vi "Escritura_Ingen.vi"(10 "Entrada_Variables":u16[](array[numeric])) -> (2 "Escritura_Variabes":u16[](array[numeric]))   [LabVIEW 2017, in "Lib_Esclavo_Ingen.lvlib"]
uses:
  Lib_Esclavo_Ingen.lvlib
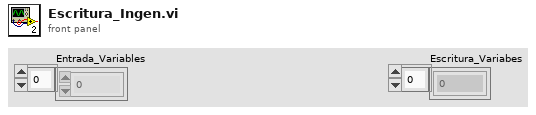
[diagram p1: front panel]
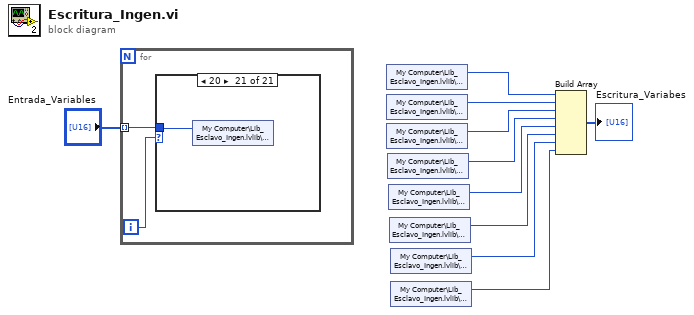
[diagram p0: block diagram]
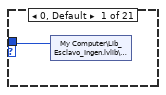
[diagram p2: hidden frame]
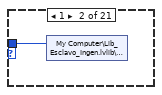
[diagram p3: hidden frame]
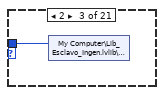
[diagram p4: hidden frame]
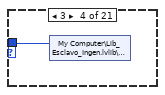
[diagram p5: hidden frame]
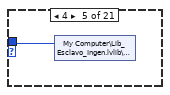
[diagram p6: hidden frame]
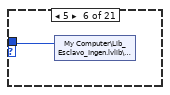
[diagram p7: hidden frame]
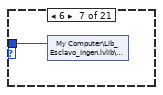
[diagram p8: hidden frame]
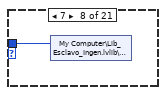
[diagram p9: hidden frame]
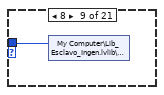
[diagram p10: hidden frame]
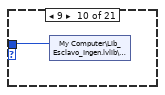
[diagram p11: hidden frame]
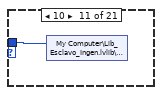
[diagram p12: hidden frame]
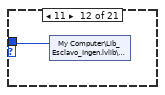
[diagram p13: hidden frame]
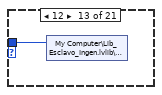
[diagram p14: hidden frame]
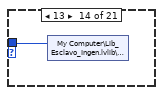
[diagram p15: hidden frame]
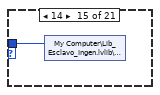
[diagram p16: hidden frame]
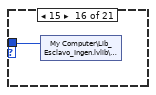
[diagram p17: hidden frame]
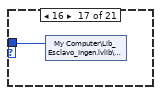
[diagram p18: hidden frame]
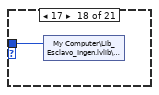
[diagram p19: hidden frame]
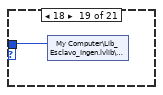
[diagram p20: hidden frame]
diagram:
  n1 = for {
    tunnel: "Entrada_Variables" -> [w11] mode=indexing
    i -> [w12]
    n2 = case shown="20" w12 {
      tunnel: w11 -> [w13 w14 w15 w16 w17 w18 w19 w20 w21 w22 w23 w24 w25 w26 w27 w28 w29 w30 w31 w32 w33]
      frame 0, Default {
        n3 = shared-variable "My Computer\\Lib_Esclavo_Ingen.lvlib\\300001"(w13) -> ()  [unwired: 1 in, 1 out]
      }
      frame 1 {
        n4 = shared-variable "My Computer\\Lib_Esclavo_Ingen.lvlib\\300002"(w14) -> ()  [unwired: 1 in, 1 out]
      }
      frame 2 {
        n5 = shared-variable "My Computer\\Lib_Esclavo_Ingen.lvlib\\300003"(w15) -> ()  [unwired: 1 in, 1 out]
      }
      frame 3 {
        n6 = shared-variable "My Computer\\Lib_Esclavo_Ingen.lvlib\\300004"(w16) -> ()  [unwired: 1 in, 1 out]
      }
      frame 4 {
        n7 = shared-variable "My Computer\\Lib_Esclavo_Ingen.lvlib\\300005"(w17) -> ()  [unwired: 1 in, 1 out]
      }
      frame 5 {
        n8 = shared-variable "My Computer\\Lib_Esclavo_Ingen.lvlib\\300006"(w18) -> ()  [unwired: 1 in, 1 out]
      }
      frame 6 {
        n9 = shared-variable "My Computer\\Lib_Esclavo_Ingen.lvlib\\300007"(w19) -> ()  [unwired: 1 in, 1 out]
      }
      frame 7 {
        n10 = shared-variable "My Computer\\Lib_Esclavo_Ingen.lvlib\\300008"(w20) -> ()  [unwired: 1 in, 1 out]
      }
      frame 8 {
        n11 = shared-variable "My Computer\\Lib_Esclavo_Ingen.lvlib\\300009"(w21) -> ()  [unwired: 1 in, 1 out]
      }
      frame 9 {
        n12 = shared-variable "My Computer\\Lib_Esclavo_Ingen.lvlib\\300010"(w22) -> ()  [unwired: 1 in, 1 out]
      }
      frame 10 {
        n13 = shared-variable "My Computer\\Lib_Esclavo_Ingen.lvlib\\300011"(w23) -> ()  [unwired: 1 in, 1 out]
      }
      frame 11 {
        n14 = shared-variable "My Computer\\Lib_Esclavo_Ingen.lvlib\\300012"(w24) -> ()  [unwired: 1 in, 1 out]
      }
      frame 12 {
        n15 = shared-variable "My Computer\\Lib_Esclavo_Ingen.lvlib\\300013"(w25) -> ()  [unwired: 1 in, 1 out]
      }
      frame 13 {
        n16 = shared-variable "My Computer\\Lib_Esclavo_Ingen.lvlib\\300014"(w26) -> ()  [unwired: 1 in, 1 out]
      }
      frame 14 {
        n17 = shared-variable "My Computer\\Lib_Esclavo_Ingen.lvlib\\300015"(w27) -> ()  [unwired: 1 in, 1 out]
      }
      frame 15 {
        n18 = shared-variable "My Computer\\Lib_Esclavo_Ingen.lvlib\\300016"(w28) -> ()  [unwired: 1 in, 1 out]
      }
      frame 16 {
        n19 = shared-variable "My Computer\\Lib_Esclavo_Ingen.lvlib\\300017"(w29) -> ()  [unwired: 1 in, 1 out]
      }
      frame 17 {
        n20 = shared-variable "My Computer\\Lib_Esclavo_Ingen.lvlib\\300018"(w30) -> ()  [unwired: 1 in, 1 out]
      }
      frame 18 {
        n21 = shared-variable "My Computer\\Lib_Esclavo_Ingen.lvlib\\300019"(w31) -> ()  [unwired: 1 in, 1 out]
      }
      frame 19 {
        n22 = shared-variable "My Computer\\Lib_Esclavo_Ingen.lvlib\\300020"(w32) -> ()  [unwired: 1 in, 1 out]
      }
      frame 20 {
        n23 = shared-variable "My Computer\\Lib_Esclavo_Ingen.lvlib\\300021"(w33) -> ()  [unwired: 1 in, 1 out]
      }
    }
  }
  n24 = shared-variable "My Computer\\Lib_Esclavo_Ingen.lvlib\\300022"() -> (w9:u16)  [unwired: 1 in, 1 out]
  n25 = shared-variable "My Computer\\Lib_Esclavo_Ingen.lvlib\\300023"() -> (w8:u16)  [unwired: 1 in, 1 out]
  n26 = shared-variable "My Computer\\Lib_Esclavo_Ingen.lvlib\\300024"() -> (w7:u16)  [unwired: 1 in, 1 out]
  n27 = shared-variable "My Computer\\Lib_Esclavo_Ingen.lvlib\\300025"() -> (w6:u16)  [unwired: 1 in, 1 out]
  n28 = shared-variable "My Computer\\Lib_Esclavo_Ingen.lvlib\\300026"() -> (w5:u16)  [unwired: 1 in, 1 out]
  n29 = shared-variable "My Computer\\Lib_Esclavo_Ingen.lvlib\\300027"() -> (w4:u16)  [unwired: 1 in, 1 out]
  n30 = shared-variable "My Computer\\Lib_Esclavo_Ingen.lvlib\\300028"() -> (w3:u16)  [unwired: 1 in, 1 out]
  n31 = shared-variable "My Computer\\Lib_Esclavo_Ingen.lvlib\\300029"() -> (w2:u16)  [unwired: 1 in, 1 out]
  n32 = Build Array(w9, w8, w7, w6, w5, w4, w3, w2) -> (→"Escritura_Variabes":u16[])
